vi "Data History - Oldest time to plot truncator.vi"(10 "Oldest Time To Plot":dbl, 11 "Full History Data":T2={"Timestamps"=[3461626102.0641413, 3461626102.7581415, 3461626102.9891415, 3461626103.2071414, 3461626103.4211416, 3461626103.6501417, 3461626103.8781414, 3461626104.1031413, 3461626104.3301415, 3461626104.5551414, 3461626104.8041415, 3461626105.0191417, 3461626105.5291414, 3461626105.8021417, 3461626106.0461416, 3461626106.3151417, 3461626106.5251417, 3461626106.7371416, 3461626106.9521413, 3461626107.1641417, 3461626107.3731413, 3461626107.5821414, 3461626107.7931414, 3461626108.0051417, 3461626108.2231417, 3461626108.4361415, 3461626108.6481414, 3461626108.8591413, 3461626109.0721416, 3461626109.2951417, 3461626109.5091414, 3461626109.7281413, 3461626109.9551415, 3461626110.1791415, 3461626110.3911414, 3461626110.6091413, 3461626110.8251414, 3461626111.0471416, 3461626111.2561417, 3461626111.4861417, 3461626111.7061415, 3461626111.9191413, 3461626112.1411414, 3461626112.3661413, 3461626112.5801415, 3461626112.8021417, 3461626113.0231414, 3461626113.2421417, 3461626113.4641414, 3461626113.6861415, 3461626113.9061413, 3461626114.1501417, 3461626114.3681417, 3461626114.5771413, 3461626114.8061414, 3461626115.0201416, 3461626115.2491417, 3461626115.4641414, 3461626115.6831417, 3461626115.9041414, 3461626116.1291413, 3461626116.3441415, 3461626116.5721416, 3461626116.7901416, 3461626117.0081415, 3461626117.2331414, 3461626117.4491415, 3461626117.6661415, 3461626117.8901415, 3461626118.1051416, 3461626118.3281417, 3461626118.5461416, 3461626118.7681413, 3461626118.9771414, 3461626119.2021413, 3461626119.4151416, 3461626119.6371417, 3461626119.8651414, 3461626120.0831413, 3461626120.3311415, 3461626120.5481415, 3461626120.7591414, 3461626120.9911413, 3461626121.2031417, 3461626121.4281416, 3461626121.6431413], "Values"=[nan, nan, nan, nan, nan, nan, nan, nan, nan, nan, nan, nan, nan, nan, nan, nan, nan, nan, nan, nan, nan, nan, nan, nan, nan, nan, nan, nan, nan, nan, nan, nan, nan, nan, nan, nan, nan, nan, nan, nan, nan, nan, nan, nan, nan, nan, nan, nan, nan, nan, nan, nan, nan, nan, nan, nan, nan, nan, nan, nan, nan, nan, nan, nan, nan, nan, nan, nan, nan, nan, nan, nan, nan, nan, nan, nan, nan, nan, nan, nan, nan, nan, nan, nan, nan, nan]} {"Timestamps" format="%^<%H:%M:%S%4u\n%x>T"}) -> (1 "Latest Timestamp":dbl, 2 "Latest Value":dbl, 3 "Truncated Data History":T1)   [LabVIEW 2015]
uses:
  typedefs/Data History.ctl
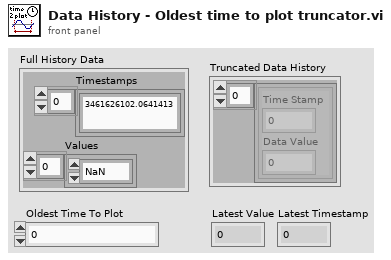
[diagram p1: front panel]
types:
  T1 = cluster{cluster{"Time Stamp":dbl, "Data Value":dbl}[]}
  T2 = typedef "Data History.ctl" = cluster{"Timestamps":dbl[], "Values":dbl[]}
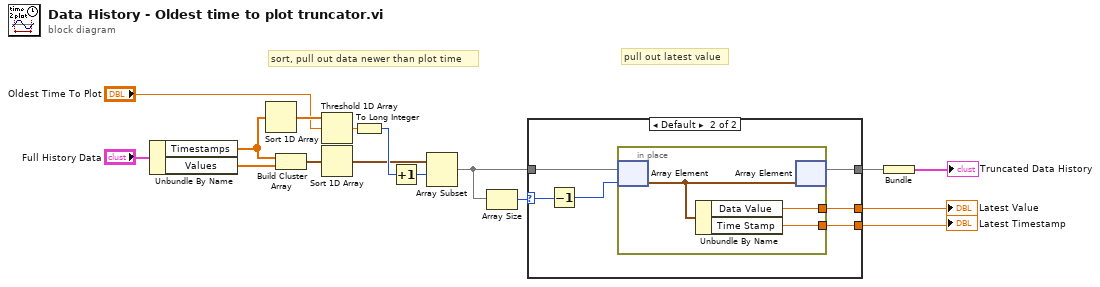
[diagram p0: block diagram]
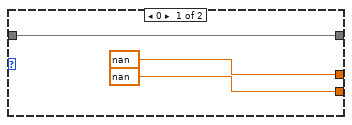
[diagram p2: hidden frame]
diagram:
  # "pull out latest value"
  # "sort, pull out data newer than plot time"
  n1 = Unbundle By Name("Full History Data") -> ("Timestamps"=w9:dbl[], "Values"=w8:dbl[])
  n2 = Sort 1D Array(array=w9) -> (sorted array=w11:dbl[])
  n3 = Build Cluster Array(w9, w8) -> (w10:cluster{"Time Stamp":dbl, "Data Value":dbl}[])
  n4 = Threshold 1D Array(2:"Oldest Time To Plot", 3:w11) -> (0:w12:dbl)  [unwired: 1 out]
  n5 = Sort 1D Array(array=w10) -> (sorted array=w13:cluster{"Time Stamp":dbl, "Data Value":dbl}[])
  n6 = To Long Integer(number=w12) -> (32bit integer=w14:i32)
  n7 = Increment(x=w14) -> (x+1=w15:i32)
  n8 = Array Subset(array=w13, index=w15) -> (w5:cluster{"Time Stamp":dbl, "Data Value":dbl}[])  [unwired: 1 in]
  n9 = Array Size(array=w5) -> (size(s)=w6:i32)
  n10 = case shown="Default" w6 {
    selector: w6 -> [_ w23]
    tunnel: w5 -> [w18 w22]
    tunnel: [nan w25] -> w4
    tunnel: [w18 w21] -> w2
    tunnel: [nan w24] -> w3
    frame 0 {
    }
    frame Default {
      n11 = Decrement(x=w23) -> (x-1=w20:i32)
      n12 = in-place {
        in-place-border: [w28] -> w25
        in-place-border: [w27] -> w24
        n13 = in-place-array #1(w22, w20) -> (w26:cluster{"Time Stamp":dbl, "Data Value":dbl})
        n14 = Unbundle By Name(w26) -> ("Data Value"=w28:dbl, "Time Stamp"=w27:dbl)
        n15 = in-place-array #1(w26) -> (w21:cluster{"Time Stamp":dbl, "Data Value":dbl}[])  [unwired: 1 out]
      }
    }
  }
  "Latest Value" <- w4
  "Latest Timestamp" <- w3
  n16 = Bundle(w2) -> (→"Truncated Data History":T1)  [unwired: 1 in]
